vi "Need_Interpolation.vi"(1 "Matrix with txt":string[][](array[string]), 2 "Number of Rows":i32) -> (0 "isNotFive?":bool)   [LabVIEW 2014]
panel:
  out "element":string
  out "index":i32
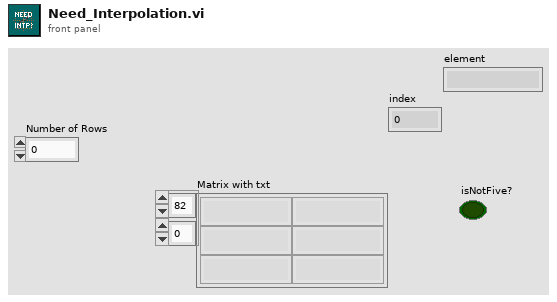
[diagram p1: front panel]
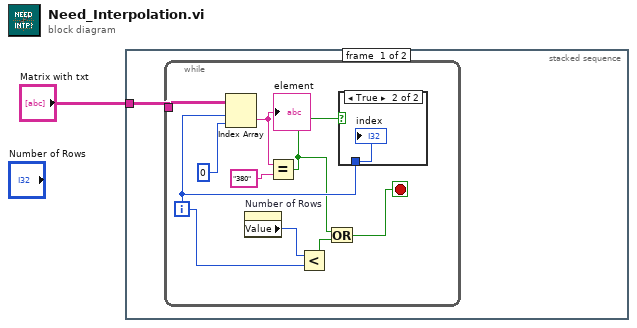
[diagram p0: block diagram]
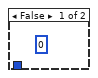
[diagram p2: hidden frame]
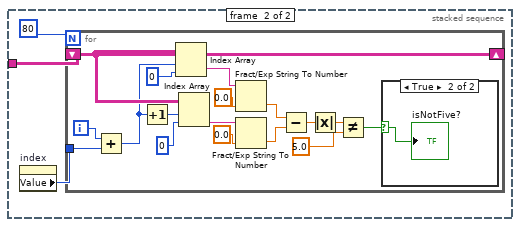
[diagram p3: hidden frame]
diagram:
  n1 = stacked-sequence {
    tunnel: "Matrix with txt" -> [w2 w15]
    frame #0 {
      n2 = while {
        tunnel: w2 -> [w11]
        i -> [w6]
        stop <- w3 stop-if-true
        n3 = Index Array(array=w11, index (row)=w6, index (col)=0 ("disabled index (col)")) -> (element=w9:string)
        "element" <- w9
        n4 = property on="Number of Rows" class="DigNum (strict)"() -> ("Value"=w7:i32)  [unwired: 2 in, 2 out]
        n5 = Equal?(x=w9, y="380") -> (x = y?=w5:bool)
        n6 = Less?(x=w7, y=w6) -> (x < y?=w4:bool)
        n7 = Or(x=w5, y=w4) -> (x .or. y?=w3:bool)
        n8 = case shown="True" w5 {
          tunnel: w6 -> [_ w12]
          frame False {
            (unwired) 0
          }
          frame True {
            "index" <- w12
          }
        }
      }
    }
    frame #1 {
      n9 = property on="index" class="DigNum (strict)"() -> ("Value"=w14:i32)  [unwired: 2 in, 2 out]
      n10 = for {
        N: 80 -> [_]
        shift-right: [w22] -> _
        shift-left: w15 -> [w22]
        tunnel: w14 -> [w16]
        i -> [w17]
        n11 = Add(x=w17, y=w16) -> (x+y=w18:i32)
        n12 = Increment(x=w18) -> (x+1=w20:i32)
        n13 = Index Array(array=w22, index (row)=w18, index (col)=0 ("disabled index (col)")) -> (element=w21:string)
        n14 = Index Array(array=w22, index (row)=w20, index (col)=0 ("disabled index (col)")) -> (element=w23:string)
        n15 = Fract/Exp String To Number(string=w21, default (0 dbl)=0.0 ("default (0 DBL)")) -> (number=w28:dbl)  [unwired: 2 in, 1 out]
        n16 = Fract/Exp String To Number(string=w23, default (0 dbl)=0.0 ("default (0 DBL)")) -> (number=w27:dbl)  [unwired: 2 in, 1 out]
        n17 = Subtract(x=w28, y=w27) -> (x-y=w26:dbl)
        n18 = Absolute Value(x=w26) -> (abs(x)=w25:dbl)
        n19 = Not Equal?(x=w25, y=5.0) -> (x != y?=w19:bool)
        n20 = case shown="True" w19 {
          selector: w19 -> [_ w33]
          frame False {
          }
          frame True {
            "isNotFive?" <- w33
          }
        }
      }
    }
  }
